vi "Joystick control (SubVI).vi"() -> (0 "G+":bool, 1 "M-":bool, 2 "M+":bool, 3 "G-":bool, 4 "Left+":bool, 5 "Right-":bool, 6 "Left-":bool, 7 "Right+":bool)   [LabVIEW 2017]
uses:
  <vilib>/myRIO/Instrument Drivers/Onboard IO/DIO/typedefs/DIO Reference.ctl
  <vilib>/myRIO/Common/Instrument Driver Framework/Utilities/typedefs/myRIO Generic Hardware Reference.ctl
  <vilib>/myRIO/Common/Instrument Driver Framework/Utilities/typedefs/Hardware Version Enum.ctl
  <vilib>/myRIO/Common/Instrument Driver Framework/Utilities/typedefs/myRIO v1.0 Reference.ctl
  <vilib>/myRIO/Common/Instrument Driver Framework/Utilities/typedefs/Generic FPGA Reference.ctl
  <vilib>/myRIO/Common/Instrument Driver Framework/myRIO v1.0/DIO/typedefs/DIO Channels List.ctl
  <vilib>/myRIO/Common/Instrument Driver Framework/myRIO v1.0/DIO/typedefs/DIO Channels Enum.ctl
  <vilib>/userdefined/High Color/nirio_resource_hc.ctl
  <vilib>/myRIO/Common/Instrument Driver Framework/Utilities/vis/Is FPGA Ref Available.vi
  <vilib>/myRIO/Common/Instrument Driver Framework/myRIO v1.0/DIO/vis/myRIO v1.1 Open DIO.vi
  <vilib>/myRIO/Instrument Drivers/Onboard IO/DIO/vis/Write.vi
  <vilib>/myRIO/Common/Instrument Driver Framework/Utilities/vis/Validate Channels.vi
  <vilib>/myRIO/Common/Instrument Driver Framework/myRIO v1.0/DIO/vis/myRIO v1.0 Reserve DIO.vi
  <vilib>/myRIO/Common/Instrument Driver Framework/myRIO v1.0/Resource Manager/vis/myRIO v1.0 Reserve Channel List.vi
  <vilib>/myRIO/Common/Instrument Driver Framework/myRIO v1.0/DIO/vis/myRIO v1.0 Build MUX Configuration DIO.vi
  <vilib>/myRIO/Common/Instrument Driver Framework/myRIO v1.0/Resource Manager/vis/myRIO v1.0 Reserve Channel.vi
  <vilib>/myRIO/Common/Instrument Driver Framework/myRIO v1.0/Resource Manager/vis/myRIO v1.0 Unreserve Channel.vi
  <vilib>/myRIO/Common/Instrument Driver Framework/myRIO v1.0/Resource Manager/vis/myRIO v1.0 Create Configuration List.vi
  <vilib>/myRIO/Common/Instrument Driver Framework/myRIO v1.0/Resource Manager/vis/myRIO v1.0 Build Mutex Name.vi
  <vilib>/Utility/VariantDataType/GetNumericInfo.vi
  <vilib>/Utility/error.llb/Error Cluster From Error Code.vi
  <vilib>/myRIO/Common/Instrument Driver Framework/myRIO v1.0/myRIO v1.1 Open.vi
  <vilib>/myRIO/Common/Instrument Driver Framework/Utilities/vis/IO Manager.vi
  <vilib>/myRIO/Common/Instrument Driver Framework/Utilities/vis/Configuration Manager.vi
  <vilib>/myRIO/Common/Instrument Driver Framework/myRIO v1.0/Resource Manager/vis/myRIO v1.0 Configure IO.vi
  <vilib>/myRIO/Common/Instrument Driver Framework/myRIO v1.0/myRIO v1.0 Close.vi
  <vilib>/myRIO/Common/Instrument Driver Framework/myRIO v1.0/DIO/vis/myRIO v1.0 Write DIO.vi
  <vilib>/myRIO/Express VI/Onboard Devices/LED/LED Express VI.xnode
  <vilib>/myRIO/Instrument Drivers/Onboard IO/DIO/vis/myRIO DIO Open.xnode
  <vilib>/myRIO/Instrument Drivers/Onboard IO/DIO/DIO.lvlib
panel:
  out "update connection":bool
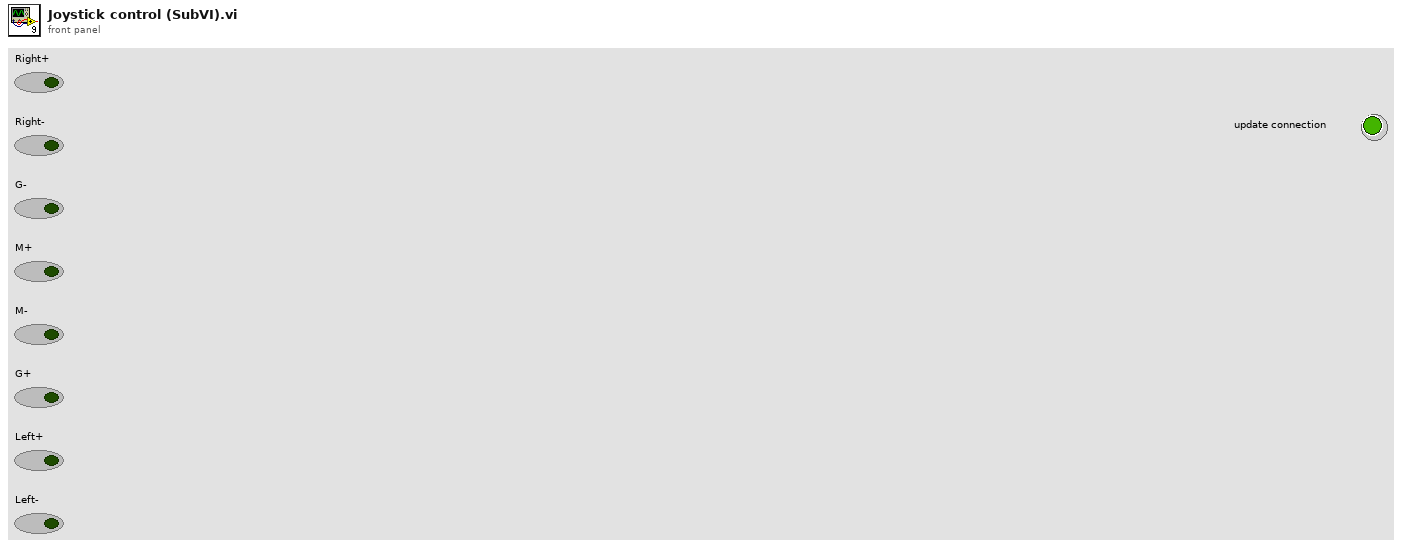
[diagram p1: front panel]
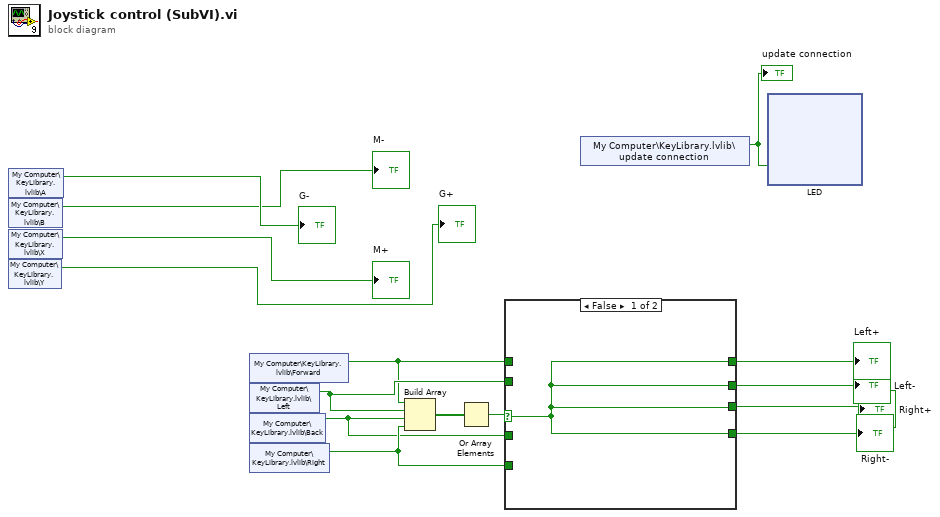
[diagram p0: block diagram]
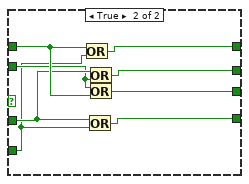
[diagram p2: hidden frame]
diagram:
  n1 = shared-variable "My Computer\\KeyLibrary.lvlib\\A"() -> (→"G-":bool)  [unwired: 1 in, 1 out]
  n2 = shared-variable "My Computer\\KeyLibrary.lvlib\\B"() -> (→"M-":bool)  [unwired: 1 in, 1 out]
  n3 = shared-variable "My Computer\\KeyLibrary.lvlib\\X"() -> (→"M+":bool)  [unwired: 1 in, 1 out]
  n4 = shared-variable "My Computer\\KeyLibrary.lvlib\\Y"() -> (→"G+":bool)  [unwired: 1 in, 1 out]
  n5 = shared-variable "My Computer\\KeyLibrary.lvlib\\Forward"() -> (w8:bool)  [unwired: 1 in, 1 out]
  n6 = shared-variable "My Computer\\KeyLibrary.lvlib\\Left"() -> (w10:bool)  [unwired: 1 in, 1 out]
  n7 = shared-variable "My Computer\\KeyLibrary.lvlib\\Back"() -> (w9:bool)  [unwired: 1 in, 1 out]
  n8 = shared-variable "My Computer\\KeyLibrary.lvlib\\Right"() -> (w11:bool)  [unwired: 1 in, 1 out]
  n9 = Build Array(w8, w10, w9, w11) -> (w7:bool[])
  n10 = Or Array Elements(Boolean array=w7) -> (logical OR=w6:bool)
  n11 = case shown="False" w6 {
    selector: w6 -> [w16 _]
    tunnel: w8 -> [_ w24]
    tunnel: w9 -> [_ w23]
    tunnel: w10 -> [_ w22]
    tunnel: w11 -> [_ w21]
    tunnel: [w16 w20] -> w12
    tunnel: [w16 w19] -> w13
    tunnel: [w16 w18] -> w14
    tunnel: [w16 w17] -> w15
    frame False {
    }
    frame True {
      n12 = Or(x=w24, y=w21) -> (x .or. y?=w18:bool)
      n13 = Or(x=w23, y=w21) -> (x .or. y?=w17:bool)
      n14 = Or(x=w23, y=w22) -> (x .or. y?=w19:bool)
      n15 = Or(x=w22, y=w24) -> (x .or. y?=w20:bool)
    }
  }
  "Right-" <- w15
  "Left+" <- w14
  "Left-" <- w13
  "Right+" <- w12
  n16 = shared-variable "My Computer\\KeyLibrary.lvlib\\update connection"() -> (w1:bool)  [unwired: 1 in, 1 out]
  "update connection" <- w1
  n17 = xnode "LED"("update connection"=w1) -> ()  [unwired: 1 in, 1 out]
